vi "Abort USer Event.vi"(8 "error in":errorcluster, 10 "Enum":T1) -> (0 "error out":errorcluster, 3 "user event out":refnum<user-event>)   [LabVIEW 2018]
doc: "The functional global creates, provides access to and destroys a user event."
uses:
  controls/Actions.ctl
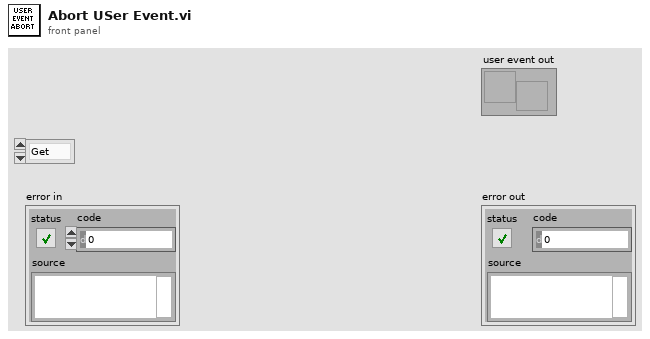
[diagram p1: front panel]
types:
  T1 = typedef "Actions.ctl" = enum16{"Get", "Create", "Destroy"}
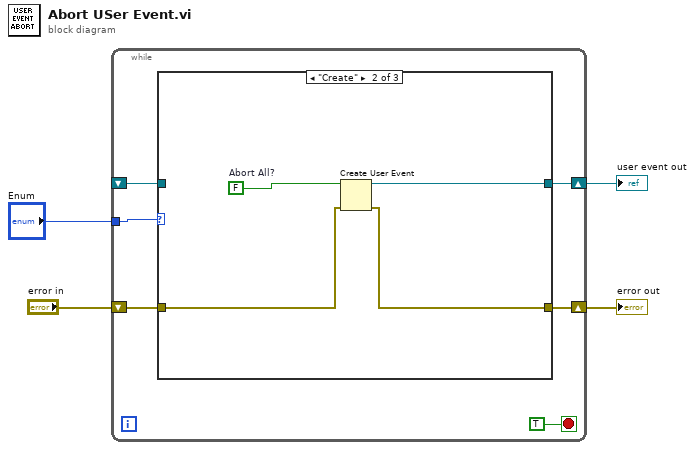
[diagram p0: block diagram]
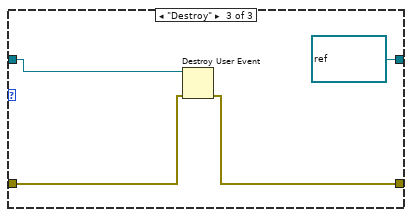
[diagram p3: hidden frame]
diagram:
  n1 = while {
    tunnel: "Enum" -> [w8]
    shift-right: [w10] -> w4
    shift-left: "error in" -> [w9]
    shift-right: [w7] -> w1
    shift-left: _ -> [w5]
    stop <- TRUE stop-if-true
    n2 = case shown="\"Create\"" w8 {
      tunnel: w9 -> [w11 w15 w18]
      tunnel: [w11 w14 w17] -> w10
      tunnel: [w12 w13 refnum<user-event> refnum ("Abort All?")] -> w7
      tunnel: w5 -> [w12 _ w19]
      frame "Get", Default {
      }
      frame "Create" {
        w16 = FALSE  # Abort All?
        n3 = Create User Event(user event datatype=w16, error in=w15) -> (user event=w13:refnum<user-event>, error out=w14:errorcluster)
      }
      frame "Destroy" {
        n4 = Destroy User Event(user event=w19, error in=w18) -> (error out=w17:errorcluster)
      }
    }
  }
  "error out" <- w4
  "user event out" <- w1
